vi "Send speed logging start notifier in imaging.vi"(11 "Setup/Logging queue element":T1={"Imaging Protocol"=enum."Live Imaging", "Number of Trials"=0, "Frame Size"=512, "# Averaged frames"=0, "Dwell time (us)"=0.0, "Index of Z-plane"=0, "Timelapse?"=FALSE, "Logging process is active"=FALSE, "Speed logging enabled"=FALSE, "tdms file ref"=refnum, "path"=path "", "Trial Number"=0, "Expected # points acquired"=FALSE, "Manually stopped"=FALSE, "Ch0 data"=[], "Ch1 data"=[], "Ref Data"=[], "Last trial"=FALSE, "Ref Dwell time (us)"=0.0, "# Ref Averaged frames"=0, "Ref X Length"=0, "Ref Y Length"=0, "Points acquired"={"Ch0 last trial"=0, "Ch1 last trial"=0, "All trials"=0}} {"Ref Dwell time (us)" format="%#.6g"; "Frame Size" items=["100X100"=100, "128X128"=128, "200X200"=200, "256X256"=256, "512X512"=512, "1024x1024"=1024, "2048x2048"=2048]; "Dwell time (us)" format="%#.6g"}) -> ()   [LabVIEW 2017]
uses:
  Typedefs/Logging queue element.ctl
  Typedefs/Imaging Protocols enum.ctl
  Typedefs/Frame Size.ctl
  Typedefs/Acquired points count.ctl
  Typedefs/Notifier Function.ctl
  Typedefs/Speed acq notifier data.ctl
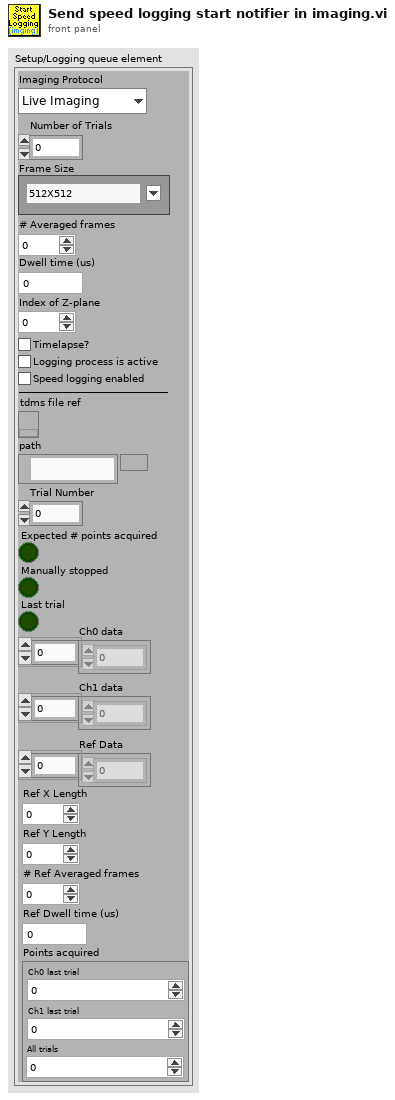
[diagram p1: front panel]
types:
  T1 = typedef "Logging queue element.ctl" = cluster{"Imaging Protocol":T2, "Number of Trials":u16, "Frame Size":T3, "# Averaged frames":u16, "Dwell time (us)":dbl, "Index of Z-plane":i32, "Timelapse?":bool, "Logging process is active":bool, "Speed logging enabled":bool, "tdms file ref":refnum<k34>, "path":path, "Trial Number":i32, "Expected # points acquired":bool, "Manually stopped":bool, "Ch0 data":u32[], "Ch1 data":u32[], "Ref Data":u32[], "Last trial":bool, "Ref Dwell time (us)":dbl, "# Ref Averaged frames":u16, "Ref X Length":u16, "Ref Y Length":u16, "Points acquired":T4}
  T2 = typedef "Imaging Protocols enum.ctl" = enum16{"AOL Z-Stack", "Motor Z Stack", "Functional Acquisition", "Single Plane Acquisition", "Volume Acquisition", "Live Imaging", "Live Plane Imaging", "Live Volume Imaging"}
  T3 = typedef "Frame Size.ctl" = u16
  T4 = typedef "Acquired points count.ctl" = cluster{"Ch0 last trial":u64, "Ch1 last trial":u64, "All trials":u64}
  T5 = typedef "Speed acq notifier data.ctl" = cluster{"Log speed data":bool, "File path":path, "Initial timestamp":timestamp}
  T6 = typedef "Notifier Function.ctl" = enum16{"Send notifier", "Wait on notification", "Release notifier"}
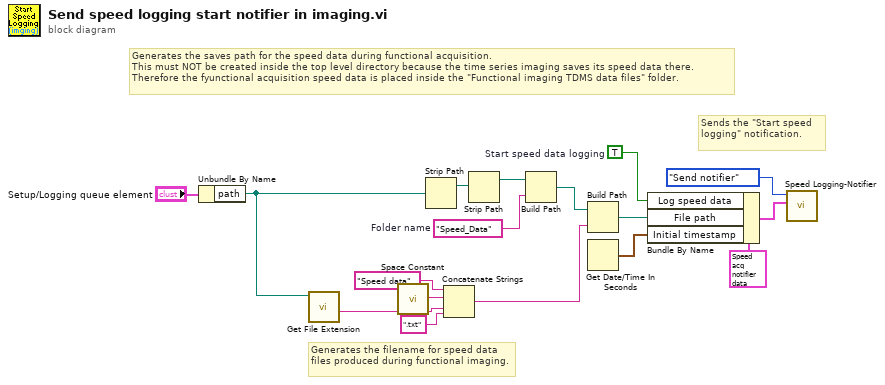
[diagram p0: block diagram]
diagram:
  w17 = TRUE  # Start speed data logging
  w14 = "Speed_Data"  # Folder name
  # "Generates the saves path for the speed data during functional acquisition.\nThis must NOT be created inside the top level directory because the time series imaging saves its speed data there.\nTherefore the fyunctional acquisition speed data is placed inside the \"Functional imaging TDMS data files\" folder."
  # "Sends the \"Start speed logging\" notification."
  # "Generates the filename for speed data files produced during functional imaging."
  n1 = Unbundle By Name("Setup/Logging queue element") -> ("path"=w2:path)
  n2 = call <vilib>:"Get File Extension.vi"("file"=w2) -> ("filename without extension"=w9:string)  [unwired: 6 in, 4 out]
  n3 = call <vilib>:"Space Constant.vi"() -> ("String"=w10:string)
  n4 = Strip Path(path=w2) -> (stripped path=w1:path)  [unwired: 1 out]
  n5 = Concatenate Strings("Speed data" ("string"), w10, w9, ".txt" ("string")) -> (w7:string)
  n6 = Strip Path(path=w1) -> (stripped path=w12:path)  [unwired: 1 out]
  n7 = Build Path(base path=w12, name or relative path=w14) -> (appended path=w13:path)
  n8 = Build Path(base path=w13, name or relative path=w7) -> (appended path=w3:path)
  n9 = Get Date/Time In Seconds() -> (seconds since 1Jan1904=w16:timestamp)
  n10 = Bundle By Name(cluster=T5 {"Log speed data"=FALSE, "File path"=path "", "Initial timestamp"=timestamp(0 s since 1904-01-01)} ("Value to send"), "Log speed data"=w17, "File path"=w3, "Initial timestamp"=w16) -> (w6:T5)
  n11 = call "Speed Logging-Notifier.vi"("Value to send"=w6, "Notifier Function"=Notifier_Function."Send notifier") -> ()  [unwired: 7 in, 3 out]
